vi "clean_up_data_tasks (SubVI).vi"(11 "data tasks":T1) -> ()   [LabVIEW 2014]
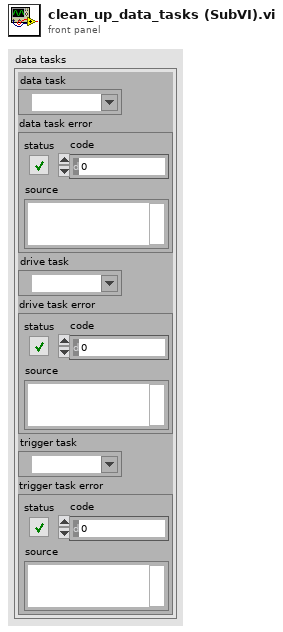
[diagram p1: front panel]
types:
  T1 = cluster{"data task":refnum<k21>, "data task error":errorcluster, "drive task":refnum<k21>, "drive task error":errorcluster, "trigger task":refnum<k21>, "trigger task error":errorcluster}
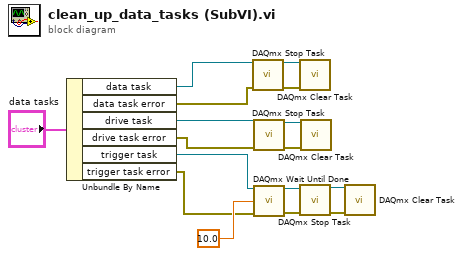
[diagram p0: block diagram]
diagram:
  n1 = Unbundle By Name("data tasks") -> ("data task"=w6:refnum<k21>, "data task error"=w5:errorcluster, "drive task"=w4:refnum<k21>, "drive task error"=w3:errorcluster, "trigger task"=w2:refnum<k21>, "trigger task error"=w1:errorcluster)
  n2 = call <vilib>:"DAQmx Stop Task.vi"("task/channels in"=w6, "error in"=w5) -> ("task out"=w8:refnum<k21>, "error out"=w9:errorcluster)  [unwired: 12 in]
  n3 = call <vilib>:"DAQmx Stop Task.vi"("task/channels in"=w4, "error in"=w3) -> ("task out"=w10:refnum<k21>, "error out"=w11:errorcluster)  [unwired: 12 in]
  n4 = call <vilib>:"DAQmx Wait Until Done.vi"("task/channels in"=w2, "timeout (sec)"=10.0, "error in"=w1) -> ("task out"=w13:refnum<k21>, "error out"=w15:errorcluster)  [unwired: 11 in]
  n5 = call <vilib>:"DAQmx Clear Task.vi"("task in"=w8, "error in"=w9) -> ()  [unwired: 13 in, 1 out]
  n6 = call <vilib>:"DAQmx Stop Task.vi"("task/channels in"=w13, "error in"=w15) -> ("task out"=w12:refnum<k21>, "error out"=w14:errorcluster)  [unwired: 12 in]
  n7 = call <vilib>:"DAQmx Clear Task.vi"("task in"=w10, "error in"=w11) -> ()  [unwired: 13 in, 1 out]
  n8 = call <vilib>:"DAQmx Clear Task.vi"("task in"=w12, "error in"=w14) -> ()  [unwired: 13 in, 1 out]
